vi "Open TDMS (All Trials).vi"(8 "error in (no error)":errorcluster, 11 "Experiment Folder":path) -> (0 "error out":errorcluster, 1 "All Files in Dir":path[](array[path]), 3 "TDMS references(All Trials)":refnum<k34>[](array[refnum]))   [LabVIEW 2017]
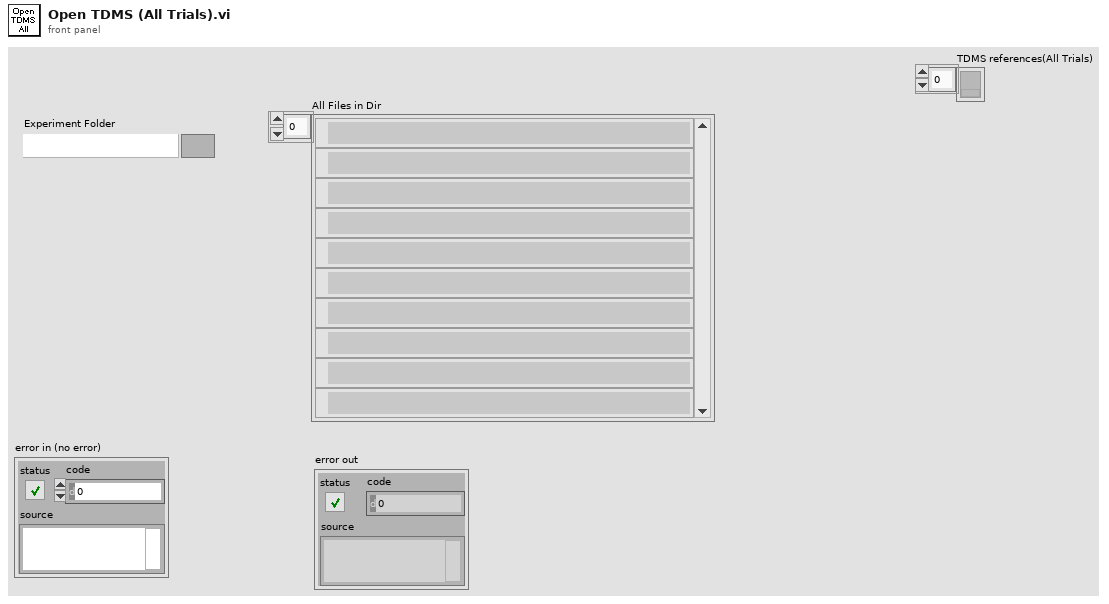
[diagram p1: front panel]
types:
  T1 = enum16{"open", "open or create", "create or replace", "create", "open (read-only)"}
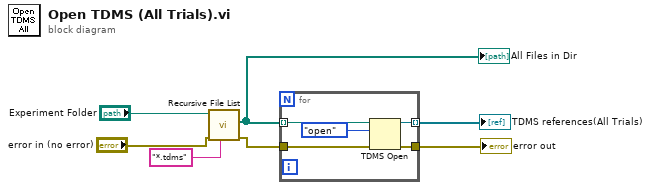
[diagram p0: block diagram]
diagram:
  n1 = call <vilib>:"Recursive File List.vi"("pattern"="*.tdms", "error in (no error)"="error in (no error)", "Folder Path"="Experiment Folder") -> ("error out"=w3:errorcluster, "All Files in Dir"=w5:path[])  [unwired: 4 in, 3 out]
  "All Files in Dir" <- w5
  n2 = for {
    tunnel: w5 -> [w12] mode=indexing
    tunnel: [w11] -> w4 mode=indexing
    tunnel: w3 -> [w9]
    tunnel: [w8] -> w1
    n3 = TDMS Open(8:w9, 10:T1."open" ("operation (0:open)"), 11:w12) -> (0:w8:errorcluster, 3:w11:refnum<k34>)  [unwired: 4 in]
  }
  "TDMS references(All Trials)" <- w4
  "error out" <- w1
